vi "VisionWrapUpNicely.vi"(11 "Refnum in":T1) -> (0 "error out":errorcluster)   [LabVIEW 2021]
uses:
  <vilib>/userDefined/High Color/IMAQdx.ctl
  <vilib>/vision/driver/NI_Vision_Acquisition_Software.lvlib
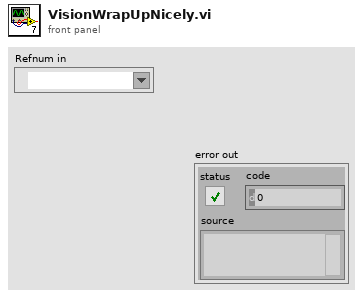
[diagram p1: front panel]
types:
  T1 = typedef "IMAQdx.ctl" = refnum<k21>
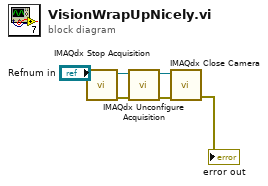
[diagram p0: block diagram]
diagram:
  n1 = call <vilib>:"IMAQdx Stop Acquisition.vi"("Session In"="Refnum in") -> ("error out"=w3:errorcluster, "Session Out"=w2:T1)  [unwired: 9 in]
  n2 = call <vilib>:"IMAQdx Unconfigure Acquisition.vi"("error in"=w3, "Session In"=w2) -> ("error out"=w5:errorcluster, "Session Out"=w4:T1)  [unwired: 8 in]
  n3 = call <vilib>:"IMAQdx Close Camera.vi"("error in"=w5, "Session In"=w4) -> ("error out"=→"error out":errorcluster)  [unwired: 9 in]
